vi "setControlIndex.vi"(8 "error in (no error)":errorcluster, 9 "VI Refnum":refnum<vi>, 10 "readBufferControlIndex":i32, 11 "UART Actor in":refnum<class "UART Actor.lvclass">) -> (0 "error out":errorcluster, 3 "UART Actor out":refnum<class "UART Actor.lvclass">)   [LabVIEW 2020, in "UART Actor.lvlib" / "UART Actor.lvclass"]
uses:
  UART Actor.lvclass
  UART Actor.lvclass/UART Actor.ctl
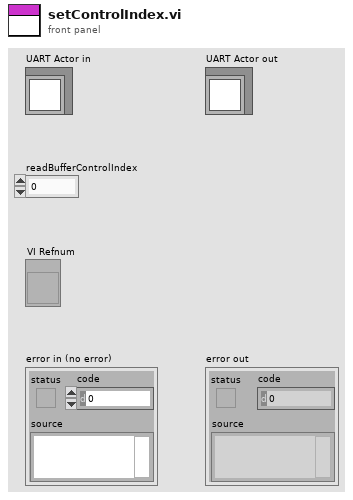
[diagram p1: front panel]
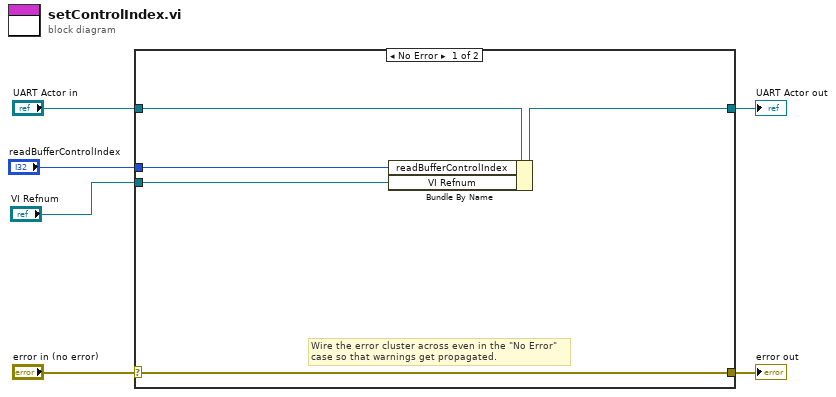
[diagram p0: block diagram]
diagram:
  n1 = case shown="No Error" "error in (no error)" {
    selector: "error in (no error)" -> [w10 w13]
    tunnel: [w10 w13] -> w5
    tunnel: [w9 w12] -> w3
    tunnel: "UART Actor in" -> [w11 w12]
    tunnel: "readBufferControlIndex" -> [w8 _]
    tunnel: "VI Refnum" -> [w7 _]
    frame No Error {
      # "Wire the error cluster across even in the \"No Error\"\ncase so that warnings get propagated."
      n2 = Bundle By Name(cluster=w11, "readBufferControlIndex"=w8, "VI Refnum"=w7) -> (w9:refnum<class "UART Actor.lvclass">)
    }
    frame Error {
    }
  }
  "error out" <- w5
  "UART Actor out" <- w3
